vi "Settings Dialog.vi"(8 "error in (no error)":errorcluster, 11 "Settings in":T1={"Hardware Configuration"={"DAQmx Channel 1"="", "DAQmx Channel 2"="", "DAQmx Channel 3"="", "Channel 1 Name"="", "Channel 2 Name"="", "Channel 3 Name"="", "Input Config Channel 1"=-1, "Input Config Channel 2"=-1, "Input Config Channel 3"=-1, "Offset Channel 1"=0.0, "Offset Channel 2"=0.0, "Offset Channel 3"=0.0, "Scale Channel 1"=0.0, "Scale Channel 2"=0.0, "Scale Channel 3"=0.0, "DAQmx Counter Channel"="", "Counter Name"="", "Sample time"=0, "Samples per second"=0.0, "Sample mode"=0, "Samples per channel"=0, "DAQmx AI Task"="", "DAQmx Counter Task"=""}, "Logging Configuration"={"Log File Base Path"=path "", "TDMS File Reference"=refnum}} {"Hardware Configuration"."Input Config Channel 3" items=["Default"=-1, "RSE"=10083, "NRSE"=10078, "Differential"=10106, "Pseudodifferential"=12529]; "Hardware Configuration"."Input Config Channel 2" items=["Default"=-1, "RSE"=10083, "NRSE"=10078, "Differential"=10106, "Pseudodifferential"=12529]; "Hardware Configuration"."Input Config Channel 1" items=["Default"=-1, "RSE"=10083, "NRSE"=10078, "Differential"=10106, "Pseudodifferential"=12529]; "Hardware Configuration"."Sample mode" items=["Hardware Timed Single Point"=12522, "Finite Samples"=10178, "Continuous Samples"=10123]}) -> (0 "error out":errorcluster, 1 "Cancelled?":bool, 2 "UI Refresh Needed?":bool, 3 "Settings out":T1={"Hardware Configuration"={"DAQmx Channel 1"="", "DAQmx Channel 2"="", "DAQmx Channel 3"="", "Channel 1 Name"="", "Channel 2 Name"="", "Channel 3 Name"="", "Input Config Channel 1"=-1, "Input Config Channel 2"=-1, "Input Config Channel 3"=-1, "Offset Channel 1"=0.0, "Offset Channel 2"=0.0, "Offset Channel 3"=0.0, "Scale Channel 1"=0.0, "Scale Channel 2"=0.0, "Scale Channel 3"=0.0, "DAQmx Counter Channel"="", "Counter Name"="", "Sample time"=0, "Samples per second"=0.0, "Sample mode"=0, "Samples per channel"=0, "DAQmx AI Task"="", "DAQmx Counter Task"=""}, "Logging Configuration"={"Log File Base Path"=path "", "TDMS File Reference"=refnum}} {"Hardware Configuration"."Input Config Channel 3" items=["Default"=-1, "RSE"=10083, "NRSE"=10078, "Differential"=10106, "Pseudodifferential"=12529]; "Hardware Configuration"."Input Config Channel 2" items=["Default"=-1, "RSE"=10083, "NRSE"=10078, "Differential"=10106, "Pseudodifferential"=12529]; "Hardware Configuration"."Input Config Channel 1" items=["Default"=-1, "RSE"=10083, "NRSE"=10078, "Differential"=10106, "Pseudodifferential"=12529]; "Hardware Configuration"."Sample mode" items=["Hardware Timed Single Point"=12522, "Finite Samples"=10178, "Continuous Samples"=10123]})   [LabVIEW 2018, in "Settings.lvlib"]
doc: "Dialog for selecting user specified settings."
uses:
  Settings.lvlib
  Settings.ctl
  Acquisition/Hardware Configuration.ctl
  Logging/Logging Configuration.ctl
  <vilib>/Utility/xml.llb/Write to XML File(string).vi
  Acquisition/Acquisition.lvlib
  Logging/Logging.lvlib
panel:
  in  "Input Config Channel 3":i32(ring)=-1 items=["Default"=-1, "RSE"=10083, "NRSE"=10078, "Differential"=10106, "Pseudodifferential"=12529]
  in  "Input Config Channel 2":i32(ring)=-1 items=["Default"=-1, "RSE"=10083, "NRSE"=10078, "Differential"=10106, "Pseudodifferential"=12529]
  in  "Input Config Channel 1":i32(ring)=-1 items=["Default"=-1, "RSE"=10083, "NRSE"=10078, "Differential"=10106, "Pseudodifferential"=12529]
  in  "Counter Channel":tag="SimDev1/ai0"
  in  "Counter Name":string="Battery Voltage"
  in  "Scale Channel 3":dbl
  in  "Scale Channel 2":dbl
  in  "Scale Channel 1":dbl
  in  "Offset Channel 3":dbl
  in  "Offset Channel 2":dbl
  in  "Offset Channel 1":dbl
  in  "Sample Mode":u16(ring)=10123 items=["Finite Samples"=10178, "Continuous Samples"=10123, "Hardware Timed Single Point"=12522]
  in  "Samples per channel":u32
  in  "Samples per second":dbl=1000.0
  in  "Sample time in ms":u32=10
  in  "Channel 3 Name":string="Brake torque"
  in  "Channel 2 Name":string="Battery Current"
  in  "Channel 1 Name":string="Battery Voltage"
  in  "Channel 3":tag="SimDev1/ai2"
  in  "Channel 2":tag="SimDev1/ai1"
  in  "Log File Path":path
  in  "Channel 1":tag="SimDev1/ai0"
  in  "Cancel Button":bool
  in  "OK Button":bool
  # "Non visible portion of dialog (needed for connector pane)."
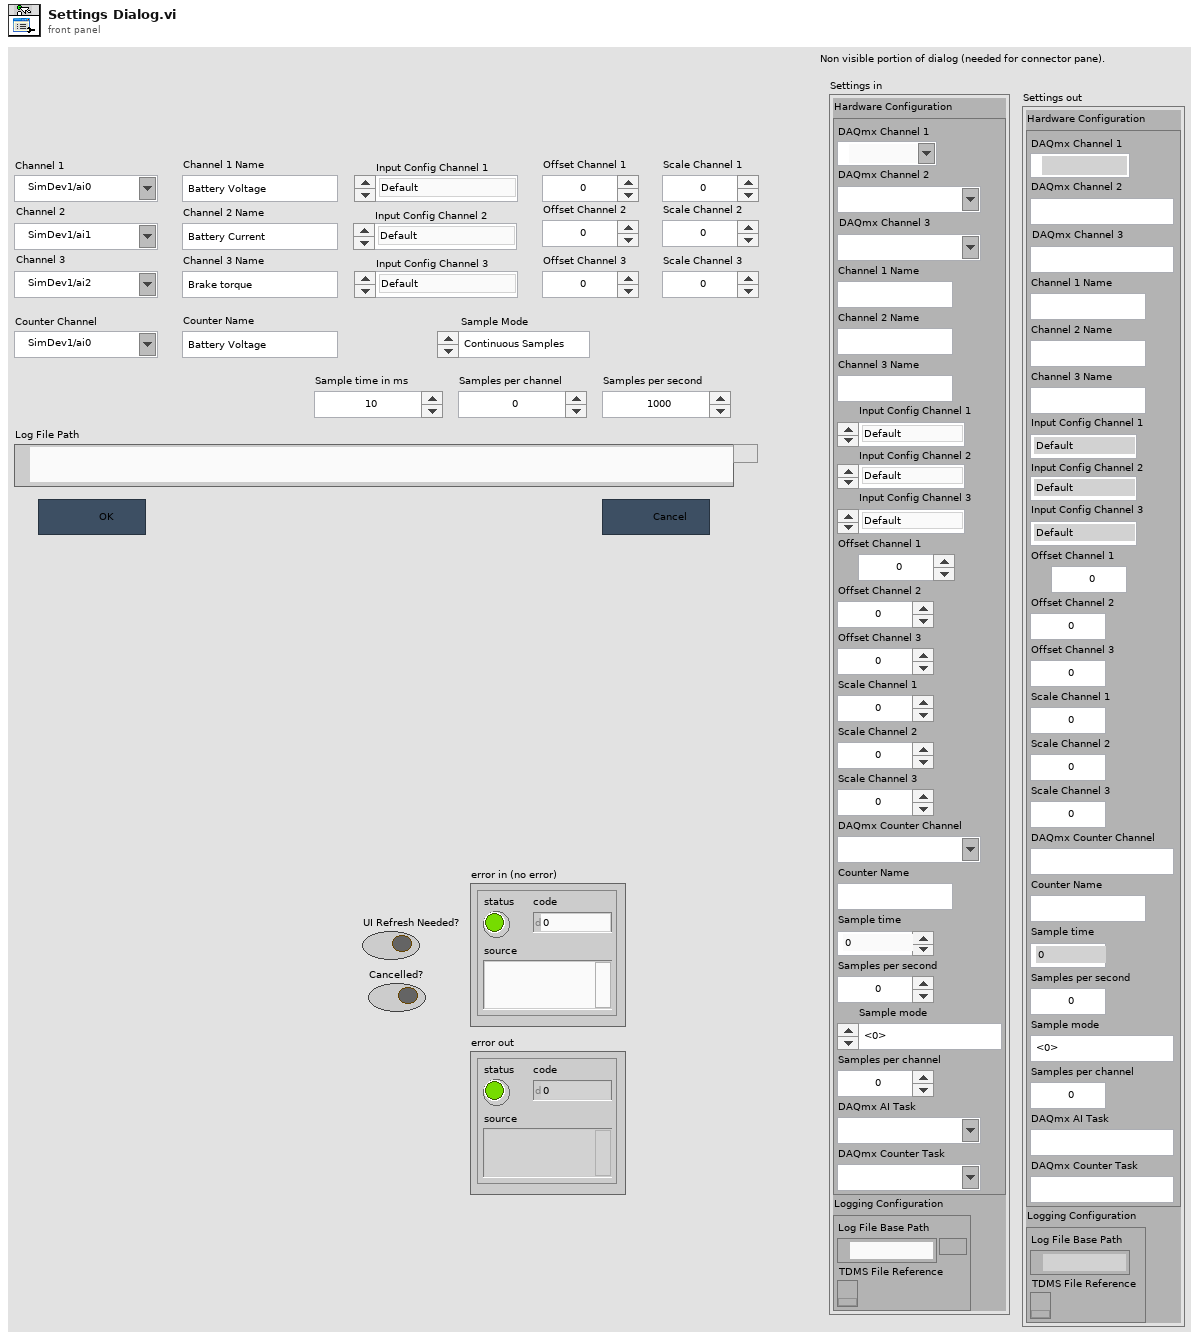
[diagram p1: front panel]
types:
  T1 = typedef "Settings.lvlib/Settings.ctl" = cluster{"Hardware Configuration":T2, "Logging Configuration":T3}
  T2 = typedef "Acquisition.lvlib/Hardware Configuration.ctl" = cluster{"DAQmx Channel 1":tag, "DAQmx Channel 2":tag, "DAQmx Channel 3":tag, "Channel 1 Name":string, "Channel 2 Name":string, "Channel 3 Name":string, "Input Config Channel 1":i32, "Input Config Channel 2":i32, "Input Config Channel 3":i32, "Offset Channel 1":dbl, "Offset Channel 2":dbl, "Offset Channel 3":dbl, "Scale Channel 1":dbl, "Scale Channel 2":dbl, "Scale Channel 3":dbl, "DAQmx Counter Channel":tag, "Counter Name":string, "Sample time":u32, "Samples per second":dbl, "Sample mode":u16, "Samples per channel":i32, "DAQmx AI Task":refnum<k21>, "DAQmx Counter Task":refnum<k21>}
  T3 = typedef "Logging.lvlib/Logging Configuration.ctl" = cluster{"Log File Base Path":path, "TDMS File Reference":refnum<k34>}
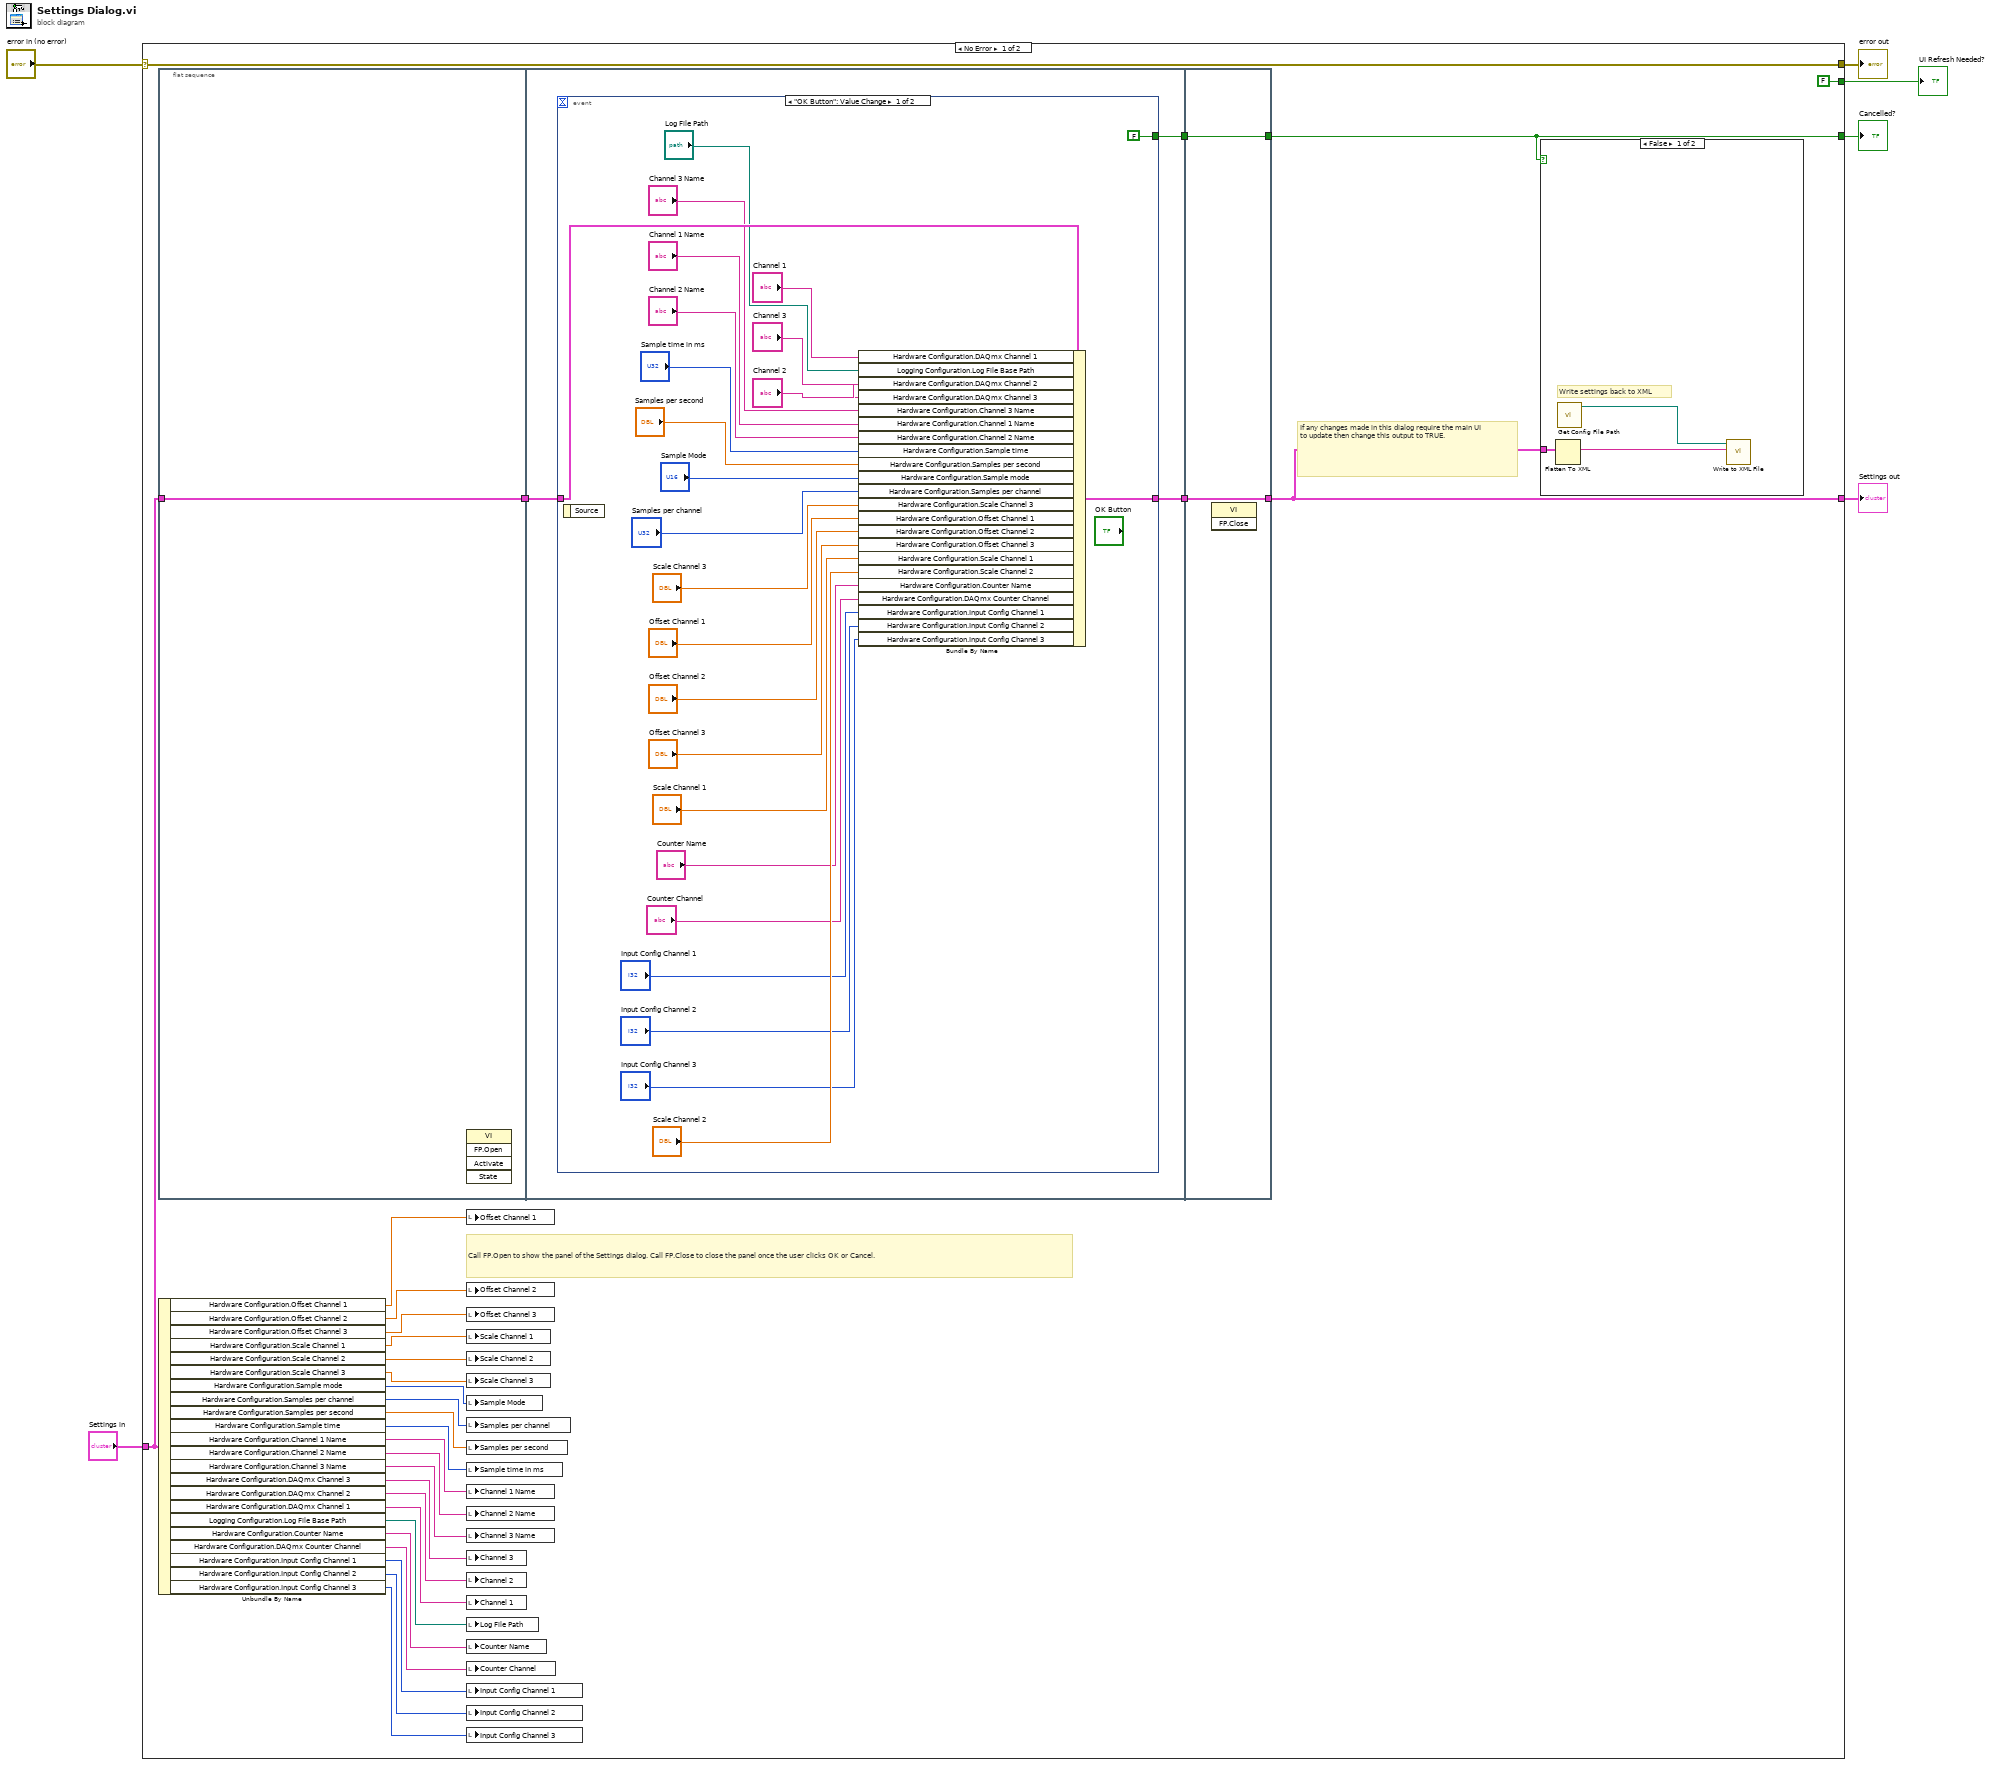
[diagram p0: block diagram]
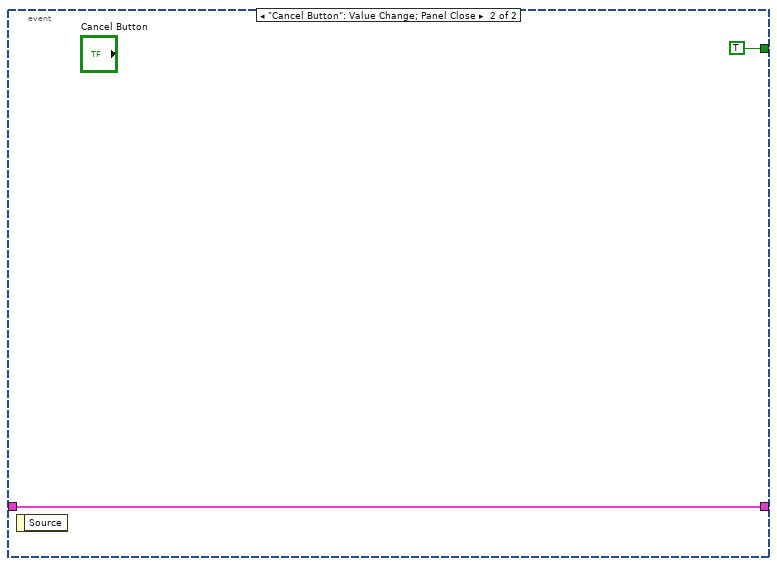
[diagram p2: hidden frame]
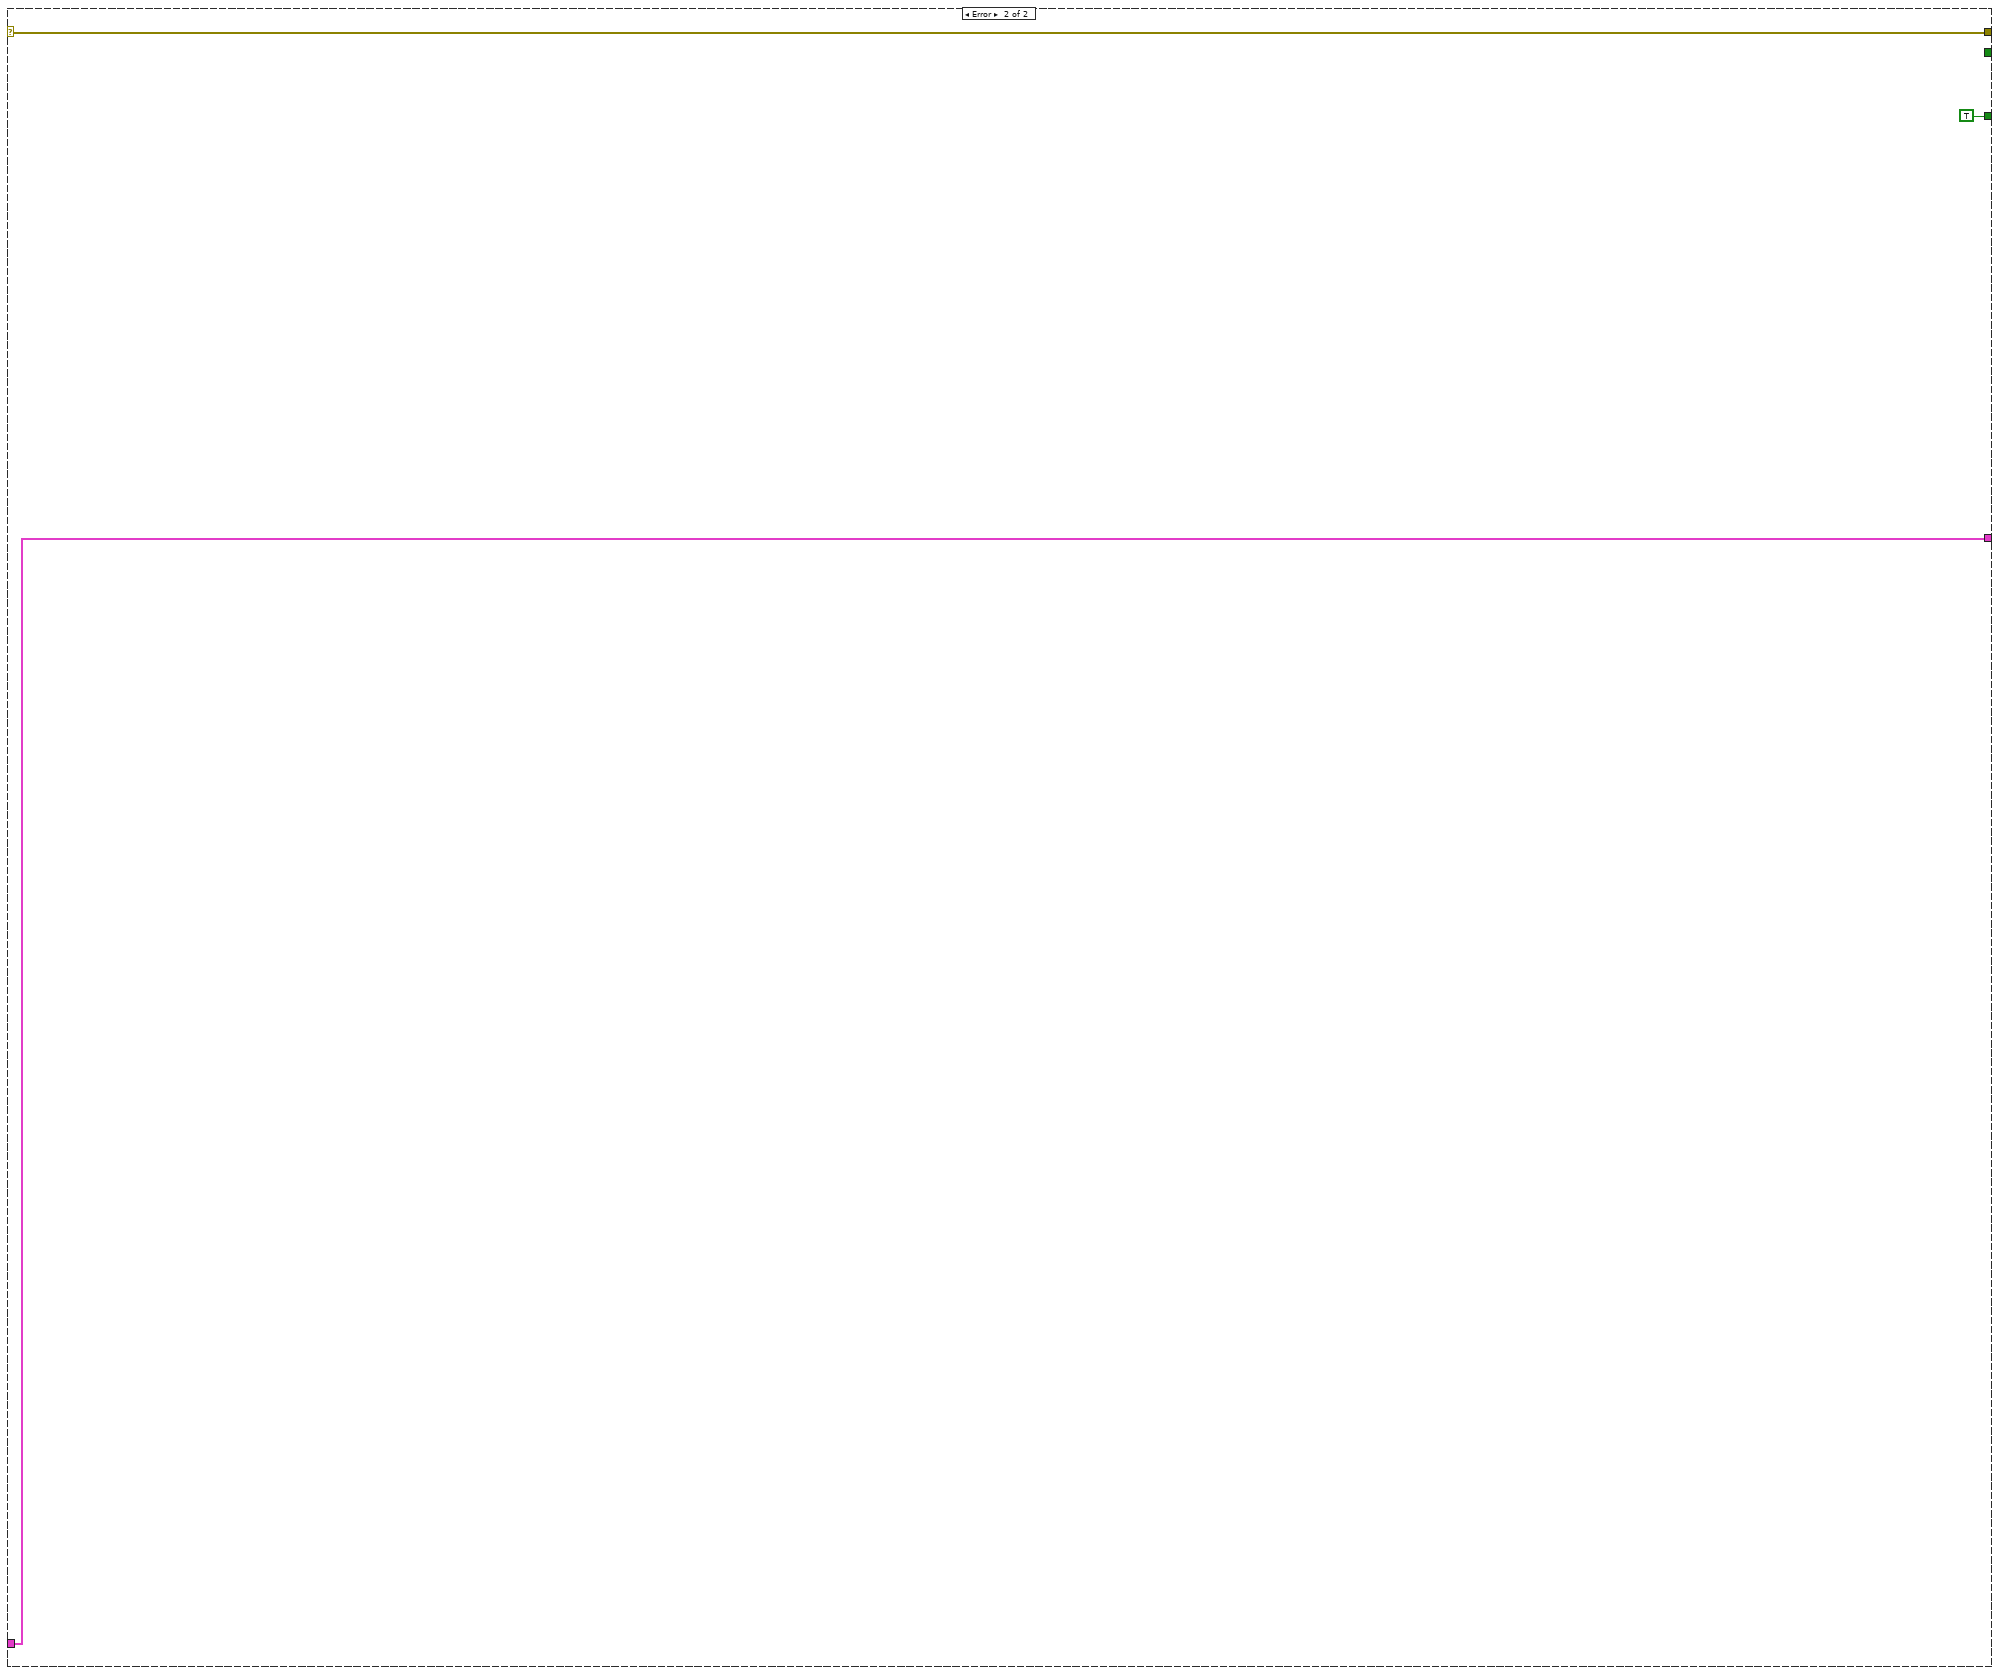
[diagram p4: hidden frame]
diagram:
  n1 = case shown="No Error" "error in (no error)" {
    selector: "error in (no error)" -> [w36 w75]
    tunnel: [w36 w75] -> w5
    tunnel: "Settings in" -> [w32 w74]
    tunnel: [w33 w74] -> w3
    tunnel: [FALSE ("UI Refresh Needed?") _] -> w2
    tunnel: [w34 TRUE ("UI Refresh Needed?")] -> w1
    frame No Error {
      # "Call FP.Open to show the panel of the Settings dialog. Call FP.Close to close the panel once the user clicks OK or Cancel."
      # "If any changes made in this dialog require the main UI to update then change this output to TRUE."
      n2 = flat-sequence {
        tunnel: w32 -> [w37]
        tunnel: [w37] -> w29
        tunnel: w29 -> [w38]
        tunnel: [w40] -> w28
        tunnel: [w39] -> w27
        tunnel: [w68] -> w33
        tunnel: [w69] -> w34
        tunnel: w28 -> [w69]
        tunnel: w27 -> [w68]
        frame #0 {
          n3 = invoke class="VI" method="FP.Open"() -> ()  [unwired: 5 in, 5 out]
        }
        frame #1 {
          n4 = event shown="[0] \"OK Button\": Value Change" {
            selector: _ -> [_ _]
            dyn-events: _ -> [_ _]
            timeout: _ -> [_ _]
            tunnel: [w63 w67] -> w39
            tunnel: w38 -> [w64 w67]
            tunnel: [FALSE ("UI Refresh Needed?") TRUE ("UI Refresh Needed?")] -> w40
            event "OK Button": Value Change {
              n5 = event-data() -> ()  [unwired: 1 in, 1 out]
              n6 = Bundle By Name(cluster=w64, "Hardware Configuration.DAQmx Channel 1"="Channel 1", "Logging Configuration.Log File Base Path"="Log File Path", "Hardware Configuration.DAQmx Channel 2"="Channel 2", "Hardware Configuration.DAQmx Channel 3"="Channel 3", "Hardware Configuration.Channel 3 Name"="Channel 3 Name", "Hardware Configuration.Channel 1 Name"="Channel 1 Name", "Hardware Configuration.Channel 2 Name"="Channel 2 Name", "Hardware Configuration.Sample time"="Sample time in ms", "Hardware Configuration.Samples per second"="Samples per second", "Hardware Configuration.Sample mode"="Sample Mode", "Hardware Configuration.Samples per channel"="Samples per channel", "Hardware Configuration.Scale Channel 3"="Scale Channel 3", "Hardware Configuration.Offset Channel 1"="Offset Channel 1", "Hardware Configuration.Offset Channel 2"="Offset Channel 2", "Hardware Configuration.Offset Channel 3"="Offset Channel 3", "Hardware Configuration.Scale Channel 1"="Scale Channel 1", "Hardware Configuration.Scale Channel 2"="Scale Channel 2", "Hardware Configuration.Counter Name"="Counter Name", "Hardware Configuration.DAQmx Counter Channel"="Counter Channel", "Hardware Configuration.Input Config Channel 1"="Input Config Channel 1", "Hardware Configuration.Input Config Channel 2"="Input Config Channel 2", "Hardware Configuration.Input Config Channel 3"="Input Config Channel 3") -> (w63:T1)
            }
            event "Cancel Button": Value Change; Panel Close {
              n7 = event-data() -> ()  [unwired: 1 in, 1 out]
            }
          }
        }
        frame #2 {
          n8 = invoke class="VI" method="FP.Close"() -> ()  [unwired: 3 in, 3 out]
        }
      }
      n9 = Unbundle By Name(w32) -> ("Hardware Configuration.Offset Channel 1"=w16:dbl, "Hardware Configuration.Offset Channel 2"=w14:dbl, "Hardware Configuration.Offset Channel 3"=w17:dbl, "Hardware Configuration.Scale Channel 1"=w12:dbl, "Hardware Configuration.Scale Channel 2"=w13:dbl, "Hardware Configuration.Scale Channel 3"=w15:dbl, "Hardware Configuration.Sample mode"=w18:u16, "Hardware Configuration.Samples per channel"=w19:i32, "Hardware Configuration.Samples per second"=w20:dbl, "Hardware Configuration.Sample time"=w21:u32, "Hardware Configuration.Channel 1 Name"=w22:string, "Hardware Configuration.Channel 2 Name"=w23:string, "Hardware Configuration.Channel 3 Name"=w24:string, "Hardware Configuration.DAQmx Channel 3"=w25:tag, "Hardware Configuration.DAQmx Channel 2"=w26:tag, "Hardware Configuration.DAQmx Channel 1"=w31:tag, "Logging Configuration.Log File Base Path"=w30:path, "Hardware Configuration.Counter Name"=w10:string, "Hardware Configuration.DAQmx Counter Channel"=w11:tag, "Hardware Configuration.Input Config Channel 1"=w9:i32, "Hardware Configuration.Input Config Channel 2"=w8:i32, "Hardware Configuration.Input Config Channel 3"=w7:i32)
      n10 = local write "Offset Channel 1"(w16) -> ()
      n11 = local write "Offset Channel 2"(w14) -> ()
      n12 = local write "Offset Channel 3"(w17) -> ()
      n13 = local write "Scale Channel 1"(w12) -> ()
      n14 = local write "Scale Channel 2"(w13) -> ()
      n15 = local write "Scale Channel 3"(w15) -> ()
      n16 = local write "Sample Mode"(w18) -> ()
      n17 = local write "Samples per channel"(w19) -> ()
      n18 = local write "Samples per second"(w20) -> ()
      n19 = local write "Sample time in ms"(w21) -> ()
      n20 = local write "Channel 1 Name"(w22) -> ()
      n21 = local write "Channel 2 Name"(w23) -> ()
      n22 = local write "Channel 3 Name"(w24) -> ()
      n23 = local write "Channel 3"(w25) -> ()
      n24 = local write "Channel 2"(w26) -> ()
      n25 = local write "Channel 1"(w31) -> ()
      n26 = local write "Log File Path"(w30) -> ()
      n27 = local write "Counter Name"(w10) -> ()
      n28 = local write "Counter Channel"(w11) -> ()
      n29 = local write "Input Config Channel 1"(w9) -> ()
      n30 = local write "Input Config Channel 2"(w8) -> ()
      n31 = local write "Input Config Channel 3"(w7) -> ()
      n32 = case shown="False" w34 {
        tunnel: w33 -> [w71 _]
        frame False {
          # "Write settings back to XML"
          n33 = Flatten To XML(anything=w71) -> (xml string=w70:string)
          n34 = call "Get Config File Path.vi"() -> ("XML File Path"=w72:path)  [unwired: 10 in, 1 out]
          n35 = call-poly <vilib>:"Write to XML File.vi"("XML Input"=w70, "XML File Path"=w72) -> ()  [unwired: 7 in, 3 out]
        }
        frame True {
        }
      }
    }
    frame Error {
    }
  }
  "UI Refresh Needed?" <- w2
  "error out" <- w5
  "Settings out" <- w3
  "Cancelled?" <- w1
